vi "Example Interrupt - Interrupt Callback.vi"(4 "Interrupt":refnum<user-event>, 5 "Event Data":T1, 6 "Control Ref":refnum<k24>, 7 "Event Common Data":T2) -> ()   [LabVIEW 2010]
uses:
  C:/tf/play/labview/Tinkerforge.dll
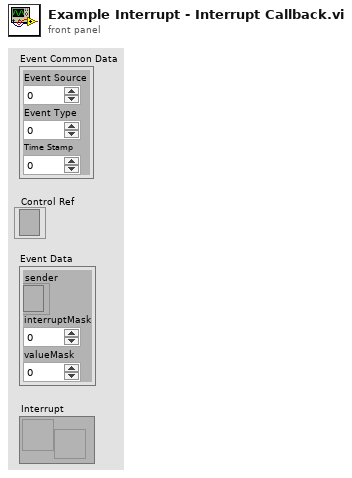
[diagram p1: front panel]
types:
  T1 = cluster{"sender":refnum<k24>, "interruptMask":i32, "valueMask":i32}
  T2 = cluster{"Event Source":i32, "Event Type":u32, "Time Stamp":u32}
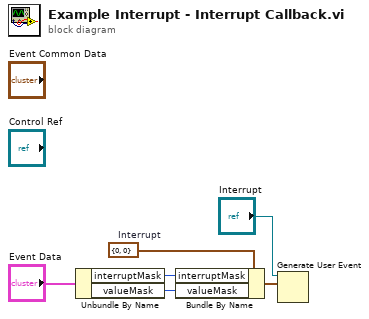
[diagram p0: block diagram]
diagram:
  w4 = cluster{"interruptMask":i32, "valueMask":i32} {"interruptMask"=0, "valueMask"=0}  # Interrupt
  n1 = Unbundle By Name("Event Data") -> ("interruptMask"=w2:i32, "valueMask"=w1:i32)
  n2 = Bundle By Name(cluster=w4, "interruptMask"=w2, "valueMask"=w1) -> (w5:cluster{"interruptMask":i32, "valueMask":i32})
  n3 = Generate User Event(user event="Interrupt", event data cluster=w5) -> ()  [unwired: 1 in, 2 out]
